vi "c_to_f.vi"(1 "C":dbl) -> (0 "F":dbl)   [LabVIEW 2013]
doc: "Hey"
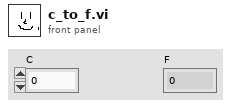
[diagram p1: front panel]
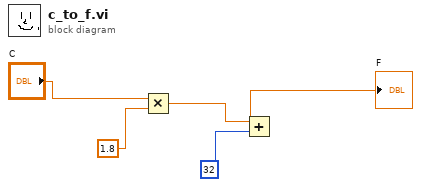
[diagram p0: block diagram]
diagram:
  n1 = Multiply(x="C", y=1.8) -> (x*y=w4:dbl)
  n2 = Add(x=w4, y=32) -> (x+y=→"F":dbl)
